vi "gu_short_path.vi"(8 "error in":errorcluster, 11 "Path":T1) -> (0 "error out":errorcluster, 3 "Short Path":T1)   [LabVIEW 2020, in "G-Unicode.lvlib"]
uses:
  G-Unicode.lvlib
  lib/g_unicode_32.dll
  Types/Encoded UTF-8 String.ctl
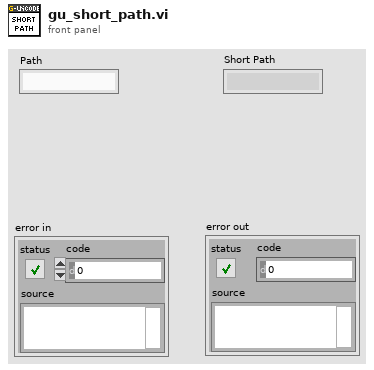
[diagram p1: front panel]
types:
  T1 = typedef "G-Unicode.lvlib/Encoded UTF-8 String.ctl" = string
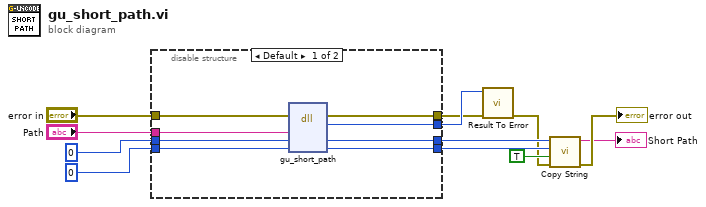
[diagram p0: block diagram]
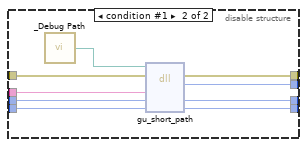
[diagram p2: hidden frame]
diagram:
  n1 = disable-structure shown="Default" {
    disable-tunnel: "Path" -> [w19 w28]
    disable-tunnel: "error in" -> [w20 w29]
    disable-tunnel: [w16 w25] -> w2
    disable-tunnel: 0 -> [w18 w27]
    disable-tunnel: i64 0 ("substring") -> [w17 w26]
    disable-tunnel: [w15 w24] -> w6
    disable-tunnel: [w14 w23] -> w5
    disable-tunnel: [w13 w22] -> w3
    frame condition #0 (active) {
      n2 = dll-call lib="C:/github/dataflowg/g-unicode/src/LabVIEW/G-Unicode/lib/g_unicode_*.*" fn="gu_short_path"(error in=w20, "path"=w19, "short_path_pointer"=w17, "short_path_length"=w18) -> (error out=w16:errorcluster, "result"=w13:i32, "short_path_pointer"=w15:i64, "short_path_length"=w14:i32)  [unwired: 3 in, 1 out]
    }
    frame condition #1 {
      n3 = call "_Debug Path.vi"() -> ("Debug Path"=w21:path)
      n4 = dll-call lib="?" fn="gu_short_path"(path in=w21, error in=w29, "path"=w28, "short_path_pointer"=w26, "short_path_length"=w27) -> (error out=w25:errorcluster, "result"=w22:i32, "short_path_pointer"=w24:i64, "short_path_length"=w23:i32)  [unwired: 2 in, 1 out]
    }
  }
  n5 = call "Result To Error.vi"("error in (no error)"=w2, "Result Code"=w3) -> ("error out"=w1:errorcluster)  [unwired: 9 in]
  n6 = call "Copy String.vi"("error in"=w1, "free (F)"=TRUE, "size"=w5, "pointer"=w6) -> ("error out"=→"error out":errorcluster, "string"=→"Short Path":string)  [unwired: 6 in]
